vi "Test Binary Config.vi"() -> ()   [LabVIEW 2021]
uses:
  Source/Abs_Types/Boolean_1D/Support/Element Type.ctl
  Source/Constants/Support/DBL_1D/Type.ctl
  Source/Abs_Types/Double Float 1D/Support/Type.ctl
  Source/Abs_Types/Boolean/Abs_Boolean.lvclass
  Source/Abs_Types/Double Float/Abs_Double Float.lvclass
  Source/Constants/Support/Bool_1D/Const_Bool_1D.lvclass
  Source/Abs_Types/Boolean_1D/Abs_Boolean_1D.lvclass
  Source/Constants/Support/DBL_1D/Const_DBL_1D.lvclass
  Source/Abs_Types/Type/Abs_Type.lvclass
  Source/Abs_Types/Double Float 1D/Abs_Double Float 1D.lvclass
  Source/Constants/Support/Bool_1D/Const_Bool_1D.lvclass/Const_Bool_1D.ctl
  Source/Constants/Support/DBL_1D/Const_DBL_1D.lvclass/Const_DBL_1D.ctl
  Source/Abs_Types/Double Float/Simple Read.vi
  Source/Abs_Types/Boolean/Simple Read.vi
  Source/Constants/Support/DBL_1D/Properties/Write Value.vi
  Source/Constants/Support/Bool_1D/Properties/Write Value.vi
  Source/Constants/Support/Bool/Bool.vi
  Source/Functions/Logic/Support/OR/Bool/Method.vi
  Source/Constants/Support/DBL/DBL.vi
  Source/Constants/Support/DBL/Const_DBL.lvclass
  Source/Constants/Support/Bool/Const_Bool.lvclass
  Source/Functions/Logic/Support/OR/Bool/OR_Bool.lvclass
panel:
  out "Value 3":T1
  out "Binary 5":string
  in  "Value 2":T2
  out "Binary":string
  out "Boolean 1D":T3[](array[typedef])
  in  "Array Value":bool[](array[boolean])
  in  "Boolean 5":bool
  out "Binary 4":string
  out "Boolean 4":bool
  in  "Boolean 3":bool
  out "Numeric 2":dbl
  in  "Numeric":dbl
  out "Binary 3":string
  in  "Boolean 2":bool
  out "Boolean":bool
  out "Binary 2":string
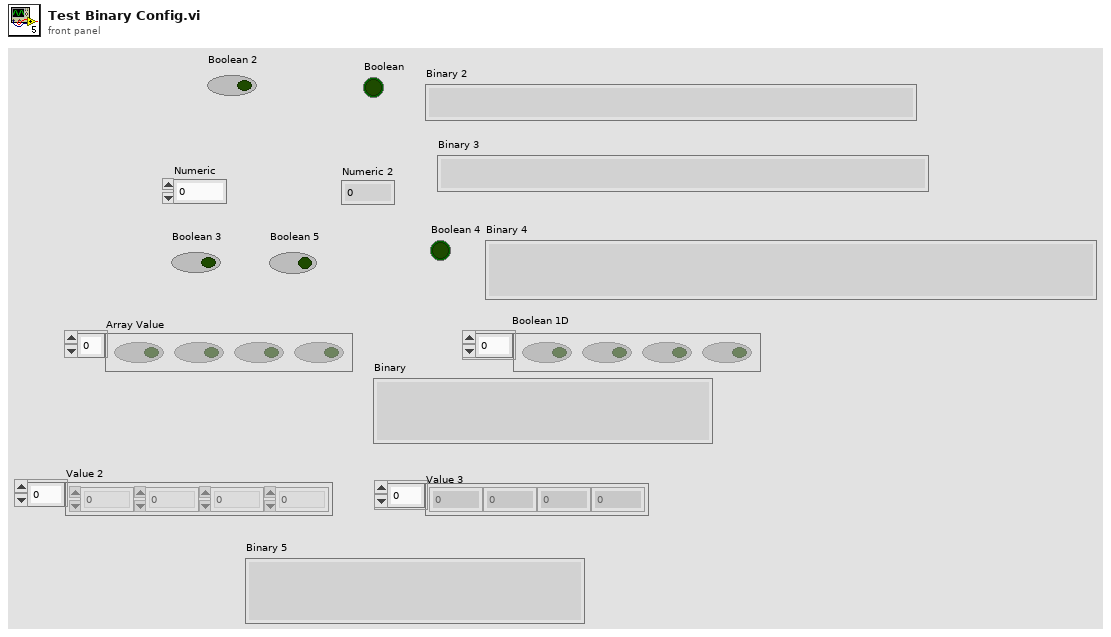
[diagram p1: front panel]
types:
  T1 = typedef "Abs_Double Float 1D.lvclass/Type.ctl" = dbl[]
  T2 = typedef "Const_DBL_1D.lvclass/Type.ctl" = dbl[]
  T3 = typedef "Abs_Boolean_1D.lvclass/Element Type.ctl" = bool
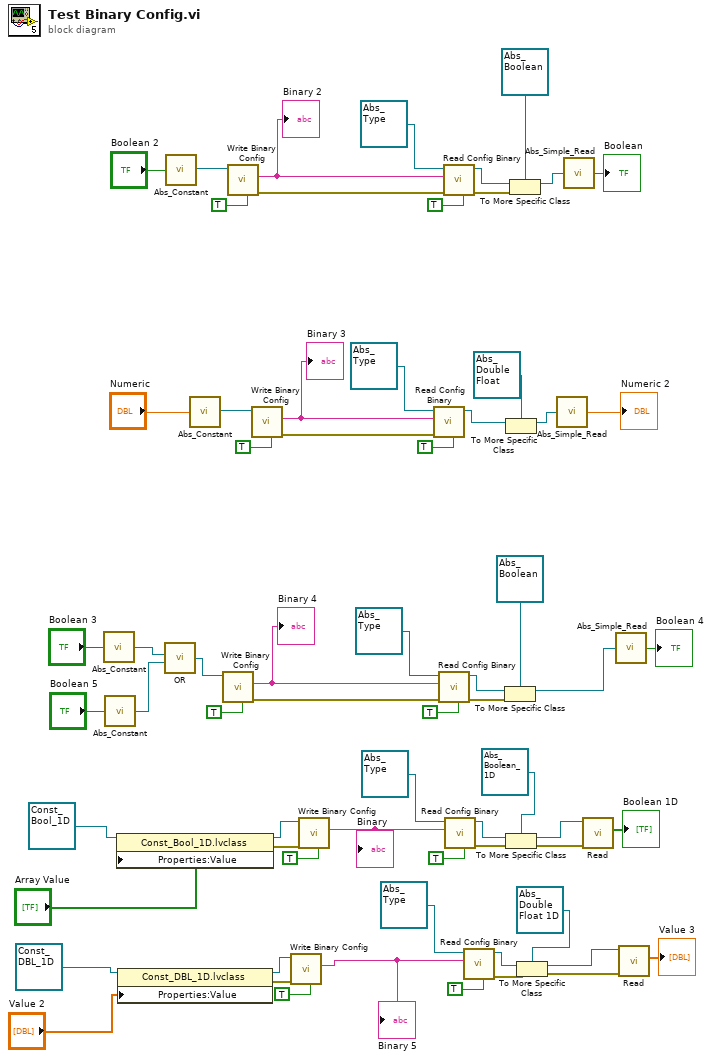
[diagram p0: block diagram]
diagram:
  n1 = call-poly "Abs_Constant.vi"("Boolean"="Boolean 3") -> ("Abs_Boolean.lvclass"=w44:refnum<class "Abs_Boolean.lvclass">)  [unwired: 4 in]
  n2 = call-poly "Abs_Constant.vi"("Boolean"="Boolean 5") -> ("Abs_Boolean.lvclass"=w42:refnum<class "Abs_Boolean.lvclass">)  [unwired: 4 in]
  n3 = property class="Const_Bool_1D.lvclass"(reference=refnum<class "Const_Bool_1D.lvclass"> refnum ("Const_Bool_1D.lvclass"), "Properties:Value"="Array Value") -> (reference out=w25:refnum<class "Const_Bool_1D.lvclass">, error out=w26:errorcluster)  [unwired: 1 in]
  n4 = property class="Const_DBL_1D.lvclass"(reference=refnum<class "Const_DBL_1D.lvclass"> refnum ("Const_DBL_1D.lvclass"), "Properties:Value"="Value 2") -> (reference out=w11:refnum<class "Const_DBL_1D.lvclass">, error out=w12:errorcluster)  [unwired: 1 in]
  n5 = call-poly "OR.vi"("B"=w42, "A"=w44) -> ("Result"=w41:refnum<class "Abs_Boolean.lvclass">)  [unwired: 4 in]
  n6 = call-poly "Abs_Constant.vi"("Boolean"="Boolean 2") -> ("Abs_Boolean.lvclass"=w66:refnum<class "Abs_Boolean.lvclass">)  [unwired: 4 in]
  n7 = call-poly "Abs_Constant.vi"("Value"="Numeric") -> ("Constant"=w39:refnum<class "Const_DBL.lvclass">)  [unwired: 4 in]
  n8 = call-dynamic "Write Binary Config.vi"("Include Class Name"=TRUE, "Abs_Type in"=w41) -> ("error out"=w53:errorcluster, "Binary"=w52:string)  [unwired: 7 in, 1 out]
  "Binary 4" <- w52
  n9 = call-dynamic "Write Binary Config.vi"("Include Class Name"=TRUE, "Abs_Type in"=w66) -> ("error out"=w56:errorcluster, "Binary"=w57:string)  [unwired: 7 in, 1 out]
  "Binary 2" <- w57
  n10 = call-dynamic "Write Binary Config.vi"("Include Class Name"=TRUE, "Const_DBL in"=w39) -> ("error out"=w33:errorcluster, "Binary"=w32:string)  [unwired: 7 in, 1 out]
  "Binary 3" <- w32
  n11 = call-dynamic "Write Binary Config.vi"("Include Class Name"=TRUE, "error in (no error)"=w12, "Const_DBL in"=w11) -> ("Binary"=w8:string)  [unwired: 6 in, 2 out]
  "Binary 5" <- w8
  n12 = call-dynamic "Write Binary Config.vi"("Include Class Name"=TRUE, "error in (no error)"=w26, "Const_Bool in"=w25) -> ("Binary"=w23:string)  [unwired: 6 in, 2 out]
  "Binary" <- w23
  n13 = call "Read Config Binary.vi"("Class Name is Included"=TRUE, "error in (no error)"=w33, "Binary"=w32, "Abs_Type in"=refnum<class "Abs_Type.lvclass"> refnum ("Abs_Type.lvclass")) -> ("Abs_Type out"=w29:refnum<class "Abs_Type.lvclass">)  [unwired: 5 in, 2 out]
  n14 = call "Read Config Binary.vi"("Class Name is Included"=TRUE, "error in (no error)"=w53, "Binary"=w52, "Abs_Type in"=refnum<class "Abs_Type.lvclass"> refnum ("Abs_Type.lvclass")) -> ("error out"=w49:errorcluster, "Abs_Type out"=w50:refnum<class "Abs_Type.lvclass">)  [unwired: 5 in, 1 out]
  n15 = call "Read Config Binary.vi"("Class Name is Included"=TRUE, "error in (no error)"=w56, "Binary"=w57, "Abs_Type in"=refnum<class "Abs_Type.lvclass"> refnum ("Abs_Type.lvclass")) -> ("error out"=w60:errorcluster, "Abs_Type out"=w59:refnum<class "Abs_Type.lvclass">)  [unwired: 5 in, 1 out]
  n16 = call "Read Config Binary.vi"("Class Name is Included"=TRUE, "Binary"=w23, "Abs_Type in"=refnum<class "Abs_Type.lvclass"> refnum ("Abs_Type.lvclass")) -> ("error out"=w22:errorcluster, "Abs_Type out"=w20:refnum<class "Abs_Type.lvclass">)  [unwired: 6 in, 1 out]
  n17 = call "Read Config Binary.vi"("Class Name is Included"=TRUE, "Binary"=w8, "Abs_Type in"=refnum<class "Abs_Type.lvclass"> refnum ("Abs_Type.lvclass")) -> ("error out"=w5:errorcluster, "Abs_Type out"=w6:refnum<class "Abs_Type.lvclass">)  [unwired: 6 in, 1 out]
  n18 = To More Specific Class(target class=refnum<class "Abs_Boolean.lvclass"> refnum ("Abs_Boolean.lvclass"), reference=w50, error in=w49) -> (specific class reference=w40:refnum<class "Abs_Boolean.lvclass">)  [unwired: 1 out]
  n19 = To More Specific Class(target class=refnum<class "Abs_Double Float.lvclass"> refnum ("Class"), reference=w29) -> (specific class reference=w35:refnum<class "Abs_Double Float.lvclass">)  [unwired: 1 in, 1 out]
  n20 = To More Specific Class(target class=refnum<class "Abs_Boolean_1D.lvclass"> refnum ("Abs_Boolean_1D.lvclass"), reference=w20, error in=w22) -> (specific class reference=w19:refnum<class "Abs_Boolean_1D.lvclass">, error out=w18:errorcluster)
  n21 = To More Specific Class(target class=refnum<class "Abs_Boolean.lvclass"> refnum ("Abs_Boolean.lvclass"), reference=w59, error in=w60) -> (specific class reference=w63:refnum<class "Abs_Boolean.lvclass">)  [unwired: 1 out]
  n22 = To More Specific Class(target class=refnum<class "Abs_Double Float 1D.lvclass"> refnum ("Abs_Double Float 1D.lvclass"), reference=w6, error in=w5) -> (specific class reference=w3:refnum<class "Abs_Double Float 1D.lvclass">, error out=w2:errorcluster)
  n23 = call-poly "Abs_Simple_Read.vi"("Class"=w35) -> ("Value"=→"Numeric 2":dbl)  [unwired: 4 in]
  n24 = call-poly "Abs_Simple_Read.vi"("Boolean in"=w63) -> ("Boolean"=→"Boolean":bool)  [unwired: 4 in]
  n25 = call-dynamic "Read.vi"("error in (no error)"=w18, "Boolean in"=w19) -> ("Boolean 1D"=→"Boolean 1D":T3[])  [unwired: 7 in, 2 out]
  n26 = call-poly "Abs_Simple_Read.vi"("Boolean in"=w40) -> ("Boolean"=→"Boolean 4":bool)  [unwired: 4 in]
  n27 = call-dynamic "Read.vi"("error in (no error)"=w2, "Double Float.lvclass_340760 in"=w3) -> ("Value"=→"Value 3":T1)  [unwired: 7 in, 2 out]
